vi "chanceof-percentage.vi"(11 "Chance of Intro":dbl) -> (3 "Present":bool)   [LabVIEW 2019]
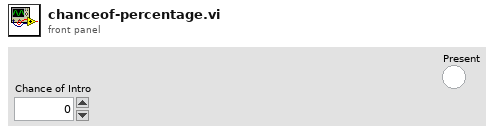
[diagram p1: front panel]
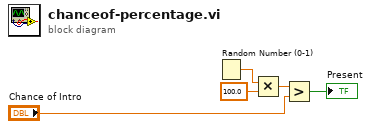
[diagram p0: block diagram]
diagram:
  n1 = Random Number (0-1)() -> (number: 0 to 1=w2:dbl)
  n2 = Multiply(x=w2, y=100.0) -> (x*y=w4:dbl)
  n3 = Greater?(x=w4, y="Chance of Intro") -> (0:→"Present":bool)
